vi "Distortion.vi"(6 "Threshold":dbl=0.45, 7 "Input":path) -> (5 "Output":path)   [LabVIEW 2012]
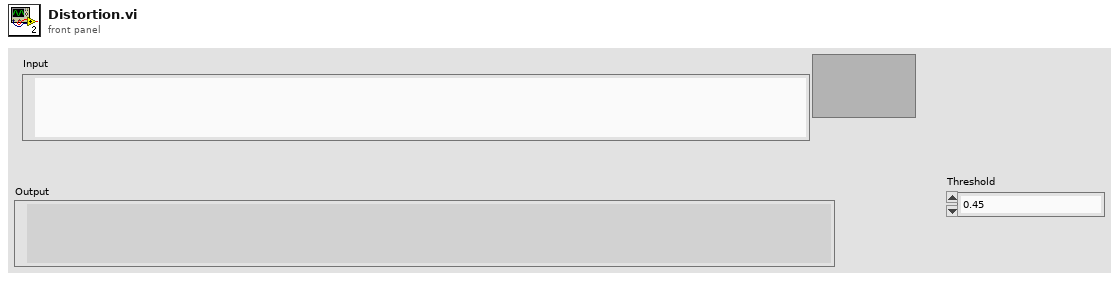
[diagram p1: front panel]
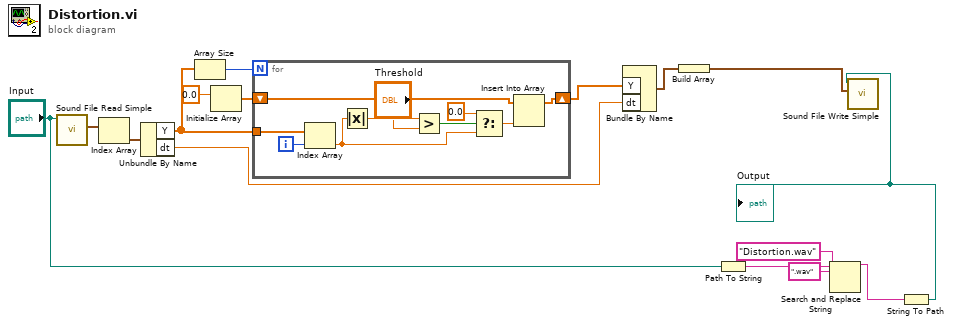
[diagram p0: block diagram]
diagram:
  n1 = call <vilib>:"Sound File Read Simple.vi"("path"="Input") -> ("data"=w16:waveform(dbl)[])  [unwired: 7 in, 3 out]
  n2 = Index Array(array=w16) -> (element=w15:waveform(dbl))  [unwired: 1 in]
  n3 = Unbundle By Name(w15) -> ("Y"=w13:dbl[], "dt"=w9:dbl)
  n4 = Array Size(array=w13) -> (size(s)=w14:i32)
  n5 = Initialize Array(0.0 ("element")) -> (w12:dbl[])  [unwired: 1 in]
  n6 = for {
    N: w14 -> [_]
    tunnel: w13 -> [w26]
    shift-right: [w17] -> w10
    shift-left: w12 -> [w22]
    i -> [w25]
    n7 = Index Array(array=w26, index=w25) -> (element=w18:dbl)
    n8 = Absolute Value(x=w18) -> (abs(x)=w24:dbl)
    n9 = Greater?(x=w24, y="Threshold") -> (0:w21:bool)
    n10 = Select(t=0.0, s=w21, f=w18) -> (s? t:f=w19:dbl)
    n11 = Insert Into Array(array=w22, new element=w19) -> (w17:dbl[])  [unwired: 1 in]
  }
  n12 = Bundle By Name("Y"=w10, "dt"=w9) -> (w8:waveform(dbl))  [unwired: 1 in]
  n13 = Build Array(w8) -> (w7:waveform(dbl)[])
  n14 = Path To String(path="Input") -> (string=w6:string)
  n15 = Search and Replace String(input string=w6, search string=".wav", replace string="Distortion.wav" ("replace string (\"\")")) -> (result string=w3:string)  [unwired: 5 in, 3 out]
  n16 = String To Path(string=w3) -> (path=w2:path)
  "Output" <- w2
  n17 = call <vilib>:"Sound File Write Simple.vi"("data"=w7, "path"=w2) -> ()  [unwired: 8 in, 2 out]
